vi "map start time tag to channel.vi"(8 "error in (no error)":errorcluster, 11 "References in":T1) -> (0 "error out":errorcluster, 3 "References out":T1)   [LabVIEW 2013, in "Shared Memory editor node.lvclass"]
uses:
  Shared Memory editor node.lvclass
  <vilib>/NI/DCAF/Tag Editor Core/Table API/Table Manager/object ref.ctl
  <vilib>/NI/DCAF/Tag Editor Core/Configuration Editor/Classes/Engine Parent/Engine Parent Editor Node.lvclass
  <vilib>/NI/DCAF/Tag Editor Core/Configuration Editor/Classes/Module editor node/module editor node.lvclass
  <vilib>/NI/Configuration Framework/serializable configuration/NISE_CEF_serializable configuration.lvclass/NISE_CEF_serializable configuration.ctl
  <vilib>/Utility/LVClass/Get LV Class Name.vi
  <vilib>/NI/Configuration Framework/error generator/NISE_error generator.vi
  <vilib>/NI/Module Execution Interface/Engine Configuration/engine configuration.lvclass
  <vilib>/NI/Configuration Framework/serializable configuration/NISE_CEF_serializable configuration.lvclass
  module/configuration/Shared Memory configuration.lvclass
  <vilib>/NI/DCAF/Tag Editor Core/Table API/Table Manager/Table Manager.lvclass
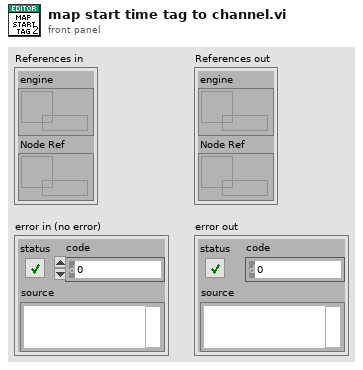
[diagram p1: front panel]
types:
  T1 = typedef "Table Manager.lvlib/Table Manager.lvclass/object ref.ctl" = cluster{"engine":refnum<data-value>, "Node Ref":refnum<data-value>}
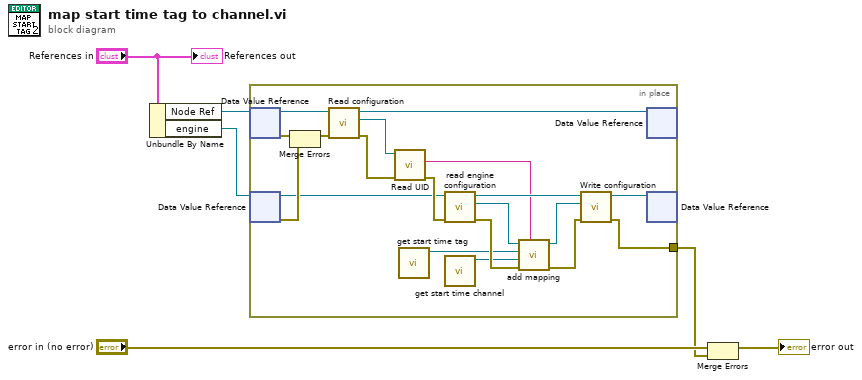
[diagram p0: block diagram]
diagram:
  n1 = Unbundle By Name("References in") -> ("Node Ref"=w3:refnum<data-value>, "engine"=w2:refnum<data-value>)
  n2 = in-place {
    in-place-border: [w10] -> w4
    n3 = in-place-dvr #1(w3) -> (w20:refnum<class "module editor node.lvclass">, w14:errorcluster)
    n4 = in-place-dvr #2(w2) -> (w11:refnum<class "Engine Parent Editor Node.lvclass">, w12:errorcluster)
    n5 = Merge Errors(w14, w12) -> (w13:errorcluster)
    n6 = call-dynamic "Read configuration.vi"("error in"=w13, "NISE_CEF_serializable node in"=w20) -> ("error out"=w18:errorcluster, "configuration"=w16:refnum<class "NISE_CEF_serializable configuration.lvclass">, "NISE_CEF_serializable node out"=w17:refnum<class "module editor node.lvclass">)  [unwired: 7 in]
    n7 = call <vilib>:"Read UID.vi"("error in"=w18, "configuration in"=w16) -> ("error out"=w15:errorcluster, "instance id"=w19:string)  [unwired: 7 in, 1 out]
    n8 = call "get start time tag.vi"() -> ("tag"=w8:refnum<class "tag descriptor.lvclass">)  [unwired: 11 in]
    n9 = call <vilib>:"read engine configuration.vi"("error in"=w15, "Engine Parent Editor Node in"=w11) -> ("error out"=w9:errorcluster, "engine configuration"=w23:refnum<class "engine configuration.lvclass">, "Engine Parent Editor Node out"=w24:refnum<class "Engine Parent Editor Node.lvclass">)  [unwired: 7 in]
    n10 = call "get start time channel.vi"() -> ("channel"=w7:refnum<class "TBM channel.lvclass">)  [unwired: 11 in]
    n11 = call <vilib>:"add mapping.vi"("owner ID"=w19, "error in"=w9, "channel"=w7, "tag descriptor"=w8, "engine configuration"=w23) -> ("error out"=w21:errorcluster, "engine configuration out"=w22:refnum<class "engine configuration.lvclass">)  [unwired: 5 in]
    n12 = call-dynamic "Write configuration.vi"("error in"=w21, "configuration"=w22, "NISE_CEF_serializable node in"=w24) -> ("error out"=w10:errorcluster, "NISE_CEF_serializable node out"=w25:refnum<class "Engine Parent Editor Node.lvclass">)  [unwired: 7 in]
    n13 = in-place-dvr #1(w17) -> ()  [unwired: 2 out]
    n14 = in-place-dvr #2(w25) -> ()  [unwired: 2 out]
  }
  n15 = Merge Errors("error in (no error)", w4) -> (→"error out":errorcluster)
  "References out" <- "References in"
